vi "Stop Module.vi"(6 "Timeout to Wait for Stop (s) (-1: no timeout)":dbl=-1.0, 8 "error in (no error)":errorcluster, 9 "Wait for Module to Stop? (F)":bool, 10 "Origin":string, 11 "TemplateAPI in":refnum<class "ExampleAPI.lvclass">) -> (0 "error out":errorcluster, 3 "TemplateAPI out":refnum<class "ExampleAPI.lvclass">)   [LabVIEW 2018, in "ExampleAPI.lvclass"]
uses:
  ExampleAPI.lvclass
  C:/Users/Phalanx/Documents/LabVIEW-Application-API-Template/src/Classes/AppControlAPI/AppControlAPI.lvclass
  AppControlAPI/AppControlAPI.lvclass/AppControlAPI.ctl
  4c94efee-2ba9-4b86-bf77-9303cd5a5534.vi
  AppControlAPI/Read AppRef.vi
  AppControlAPI/Insert In Reference Cache.vi
  AppControlAPI/Read Cache.vi
  AppControlAPI/Write Cache.vi
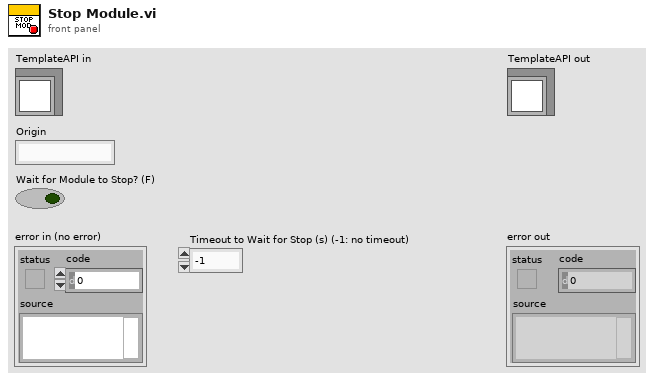
[diagram p1: front panel]
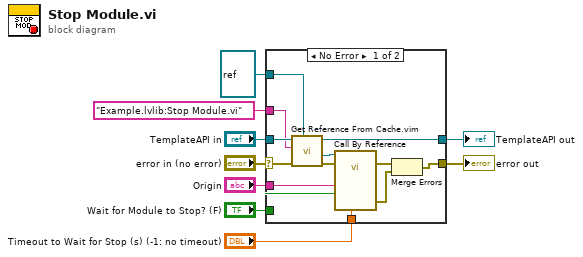
[diagram p0: block diagram]
diagram:
  n1 = case shown="No Error" "error in (no error)" {
    selector: "error in (no error)" -> [w18 w24]
    tunnel: [w15 w24] -> w8
    tunnel: [w21 w23] -> w6
    tunnel: "TemplateAPI in" -> [w22 w23]
    tunnel: "Origin" -> [w16 _]
    tunnel: "Example.lvlib:Stop Module.vi" ("VIQualifiedName") -> [w13 _]
    tunnel: refnum<vi> refnum ("type specifier VI Refnum (for type only)") -> [w12 _]
    tunnel: "Wait for Module to Stop? (F)" -> [w11 _]
    tunnel: "Timeout to Wait for Stop (s) (-1: no timeout)" -> [w10 _]
    frame No Error {
      n2 = call "Get Reference From Cache.vim"("type specifier VI Refnum (for type only)"=w12, "error in (no error)"=w18, "VIQualifiedName"=w13, "AppControlAPI in"=w22) -> ("error out"=w19:errorcluster, "VIRef"=w20:refnum<vi>, "AppControlAPI out"=w21:refnum<class "ExampleAPI.lvclass">)  [unwired: 5 in]
      n3 = call-by-ref "?"(reference=w20, error in=w19, "Timeout to Wait for Stop (s) (-1: no timeout)"=w10, "Wait for Module to Stop? (F)"=w11, "Origin"=w16) -> (error out=w17:errorcluster, 0:"error out"=w14:errorcluster)  [unwired: 8 in, 1 out]
      n4 = Merge Errors(w17, w14) -> (w15:errorcluster)
    }
    frame Error {
    }
  }
  "error out" <- w8
  "TemplateAPI out" <- w6
